vi "Autonomous Independent.vi"() -> ()   [LabVIEW 2016]
doc: "This VI is called when autonomous begins, and will automatically be terminated when autonomous ends. You can carry out timed or sensor driven robot movement independently without needing to return to the caller."
uses:
  <vilib>/Rock Robotics/WPI/ThirdParty/Sensors/Pigeon IMU/CTRE_PigeonIMU_TareType.ctl
  <vilib>/Rock Robotics/WPI/ThirdParty/CanMotor/TalonSRX/WPI_CANTalonSRX_BrakeOverride.ctl
  <vilib>/Rock Robotics/WPI/ThirdParty/CanMotor/TalonSRX/WPI_CANTalonSRX_APIControlMode.ctl
  Robot Global Data.vi
  <vilib>/Rock Robotics/Network Tables/NT Read Numeric Array.vi
  <vilib>/Rock Robotics/Network Tables/NT Write Number.vi
  <vilib>/Rock Robotics/Network Tables/NT Read String.vi
panel:
  in  "Disable Drive":bool
  in  "Norm":bool
  in  "Ms to top throttle":dbl=750.0 format="%#_13g"
  in  "Custom Sequence 2":cluster{"Values":dbl[], "Operation":u16[]}={"Values"=[0.0], "Operation"=[1000]} {"Operation" items=["Start"=0, "Drive Distance"=1, "Spin"=2, "Eject"=3, "Drive Time"=4, "Shoot Time"=5, "End"=1000, "Hold Position for ever"=1001]}
  in  "Custom Sequence 1":cluster{"Values":dbl[], "Operation":u16[]}={"Values"=[0.0], "Operation"=[1000]} {"Operation" items=["Start"=0, "Drive Distance"=1, "Spin"=2, "Eject"=3, "Drive Time"=4, "Shoot Time"=5, "End"=1000, "Hold Position for ever"=1001]}
  in  "Use Front Pannel":bool=TRUE
  in  "IZone":dbl=100.0
  in  "I":dbl=0.0125
  in  "Value to pass":dbl
  in  "Operation":i32
  in  "Start":bool
  in  "Go":bool
  in  "Case":i32
  in  "String":string="Nothing"
  in  "Rotate max throttle":dbl=0.666
  in  "Accept Error":dbl=1.0
  in  "F":dbl=0.11
  in  "P":dbl=0.0085
  in  "Acceptable Closed Loop error":dbl=0.01
  in  "Wheel Diameter":dbl=4.125
  in  "P":dbl=1.7
  in  "I":dbl
  in  "D":dbl=100.0
  in  "F":dbl=0.195
  in  "I Zone":dbl
  in  "Ramp Rate":dbl
  in  "P 2":dbl=1.7
  in  "I 2":dbl
  in  "D 2":dbl=100.0
  in  "F 2":dbl=0.195
  in  "I Zone 2":dbl
  in  "Ramp Rate 2":dbl
  # "Custom operation"
  # "Flow   Control"
  # "miscellaneous"
  # "Right"
  # "Left"
  # "Rotate"
  # "Drive Distance"
  # "Drive for time"
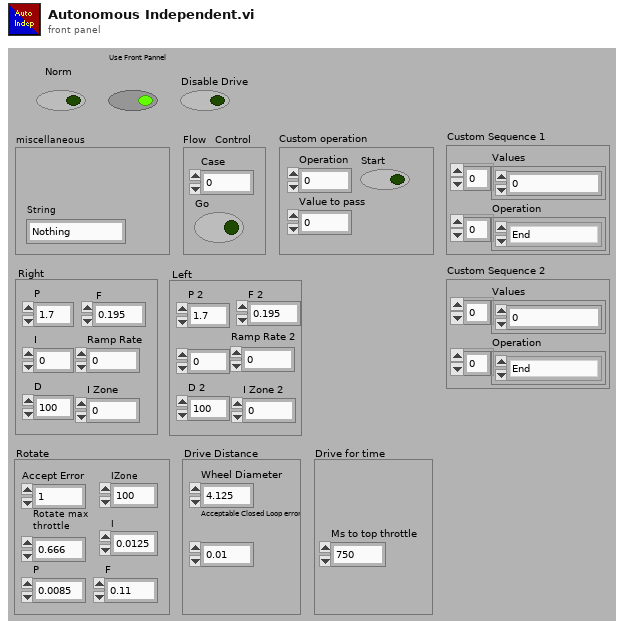
[diagram p1: front panel]
types:
  T1 = typedef "WPI_CANTalonSRX_BrakeOverride.ctl" = enum8{"No Override", "Override to Coast", "Override to Brake"}
  T2 = typedef "CTRE_PigeonIMU_TareType.ctl" = u8
  T3 = cluster{"P":dbl, "I":dbl, "D":dbl, "F":dbl, "IZone":dbl, "RampRate":dbl}
  T4 = enum16{"SOLID", "FLASH 500ms", "FLASH 1000ms", "OFF"}
  T5 = enum16{"OFF", "RED", "GREEN", "BLUE", "PURPLE", "YELLOW", "TEAL", "WHITE", "RAINBOW"}
  T6 = typedef "CTRE_PigeonIMU_DeviceRef.ctl" = cluster{"DeviceStatus":errorcluster, "Device Number":u8, "Type":T7, "Device ID":u32}
  T7 = typedef "CTRE_PigeonIMU_ConnectionType.ctl" = u32
  T8 = typedef "CTRE_PigeonIMU_GlobalStatus.ctl" = cluster{"PigeonState":T9, "FusedHeading":cluster{"Heading":dbl, "Valid?":bool, "Fusing?":bool}, "YPR":cluster{"Yaw":dbl, "Pitch":dbl, "Roll":dbl}, "Compass":cluster{"Heading":dbl, "Magnitude":dbl, "Absolute Heading":dbl}, "Accelerometer":cluster{"Biased":cluster{"X":i16, "Y":i16, "Z":i16, "Norm":i16}, "Angles":cluster{"XZ Tilt":dbl, "YZ Tilt":dbl, "XY Tilt":dbl}}, "Magnetometer":cluster{"Raw":cluster{"X":i16, "Y":i16, "Z":i16}, "Biased":cluster{"X":i16, "Y":i16, "Z":i16}}, "Gyro":cluster{"X":dbl, "Y":dbl, "Z":dbl, "Norm":dbl}, "6D Quaternian":cluster{"W":dbl, "X":dbl, "Y":dbl, "Z":dbl}, "Temp. (C)":dbl, "UpTime":u32, "StartupStatus":cluster{"ResetCount":i32, "ResetFlags":i32, "FirmwareVersion":i32, "HasReset?":bool}, "Calibration":cluster{"CurrentMode":T10, "LastCalError":i32, "CalBooting?":bool}, "CAN Error":errorcluster, "AccumGyro":cluster{"X":dbl, "Y":dbl, "Z":dbl}, "Usage Frame":u32}
  T9 = typedef "CTRE_PigeonIMU_PigeonState.ctl" = enum16{"NoComm", "Initializing", "Ready", "UserCalibration"}
  T10 = typedef "CTRE_PigeonIMU_CalibrationMode.ctl" = u16
  T11 = typedef "WPI_MotorControlDeviceRef.ctl" = cluster{"DeviceStatus":errorcluster, "Type":T12, "PWM":cluster{"PWM Channel":T13, "DeadBand":T14}, "CAN":cluster{"Device Number":u8, "SetOutput VI Ref":variant, "GetOutput VI Ref":variant, "Enable VI Ref":variant, "Disable VI Ref":variant, "Data":variant}, "Invert":bool}
  T12 = typedef "WPI_MotorControlType.ctl" = enum16{"PWM", "CAN"}
  T13 = typedef "FPGA_DIOPWMChannel.ctl" = enum8{"PWM 0", "PWM 1", "PWM 2", "PWM 3", "PWM 4", "PWM 5", "PWM 6", "PWM 7", "PWM 8", "PWM 9", "PWM MXP 0", "PWM MXP 1", "PWM MXP 2", "PWM MXP 3", "PWM MXP 4", "PWM MXP 5", "PWM MXP 6", "PWM MXP 7", "PWM MXP 8", "PWM MXP 9", "Invalid"}
  T14 = typedef "WPI_PWMDeadband.ctl" = cluster{"Name":string, "maxPositivePwm":i32, "minPositivePwm":i32, "centerPwm":i32, "maxNegativePwm":i32, "minNegativePwm":i32, "angularRange":u16}
  T15 = typedef "WPI_ServoDeviceRef.ctl" = cluster{"DeviceStatus":errorcluster, "PWM Channel":T13, "DeadBand":T14}
  T16 = typedef "WPI_CANTalonSRX_GlobalStatus.ctl" = cluster{"Applied Throttle":dbl, "Module Enabled":bool, "CAN Error":errorcluster, "Closed Loop Error":dbl, "Forward Limit Switch Closed":bool, "Reverse Limit Switch Closed":bool, "Sensor Position":dbl, "Sensor Velocity":dbl, "Current":dbl, "Sticky Fault - Over Temp":bool, "Sticky Fault - Under Voltage":bool, "Sticky Fault - Forward Limit":bool, "Sticky Fault - Reverse Limit":bool, "Sticky Fault - Forward Soft Limit":bool, "Sticky Fault - Reverse Soft Limit":bool, "Brake is Enabled":bool, "Encoder Position":dbl, "Encoder Velocity":dbl, "Encoder Index Count":dbl, "Encoder A Pin State":bool, "Encoder B Pin State":bool, "Encoder Index Pin State":bool, "Analog In":dbl, "Analog In Velocity":dbl, "Temperature (C)":dbl, "Battery Voltage":dbl, "Control 5 Is Supported":bool, "Current Profile Slot Select":dbl, "Pos Div 8":bool, "Vel Div 4":bool, "Pulse Width Position":i32, "Pulse Width Velocity":i32, "Pulse Width Rise To Rise (us)":i32, "Pulse Width Rise To Fall (us)":i32, "Mot Prof Active Is Under Run":bool, "Mot Prof Active Has Under Run":bool, "Mot Prof Active Is Last":bool, "Mot Prof Active Velocity Only":bool, "Mot Prof Active Is Valid":bool, "Mot Prof Buffer Is Full":bool, "Mot Prof Active Profile Slot Select":i32, "Mot Prof NextID":i32, "Mot Prof Count":i32, "Mot Prof Active Velocity":dbl, "Mot Prof Active Position":dbl, "Mot Prof Output Enable":i32, "UsageFrame":u32, "Motion Magic Active Trajectory":cluster{"Velocity":dbl, "Position":dbl}}
  T17 = typedef "WPI_CANTalonSRX_APIControlMode.ctl" = enum8{"Percent VBus", "Speed", "Position", "Slave", "Unchanged / Invalid", "Voltage Compensation", "Current", "Motion Profile", "Motion Magic"}
  T18 = typedef "NetComm_AllianceStation.ctl" = enum16{"Red 1", "Red 2", "Red 3", "Blue 1", "Blue 2", "Blue 3"}
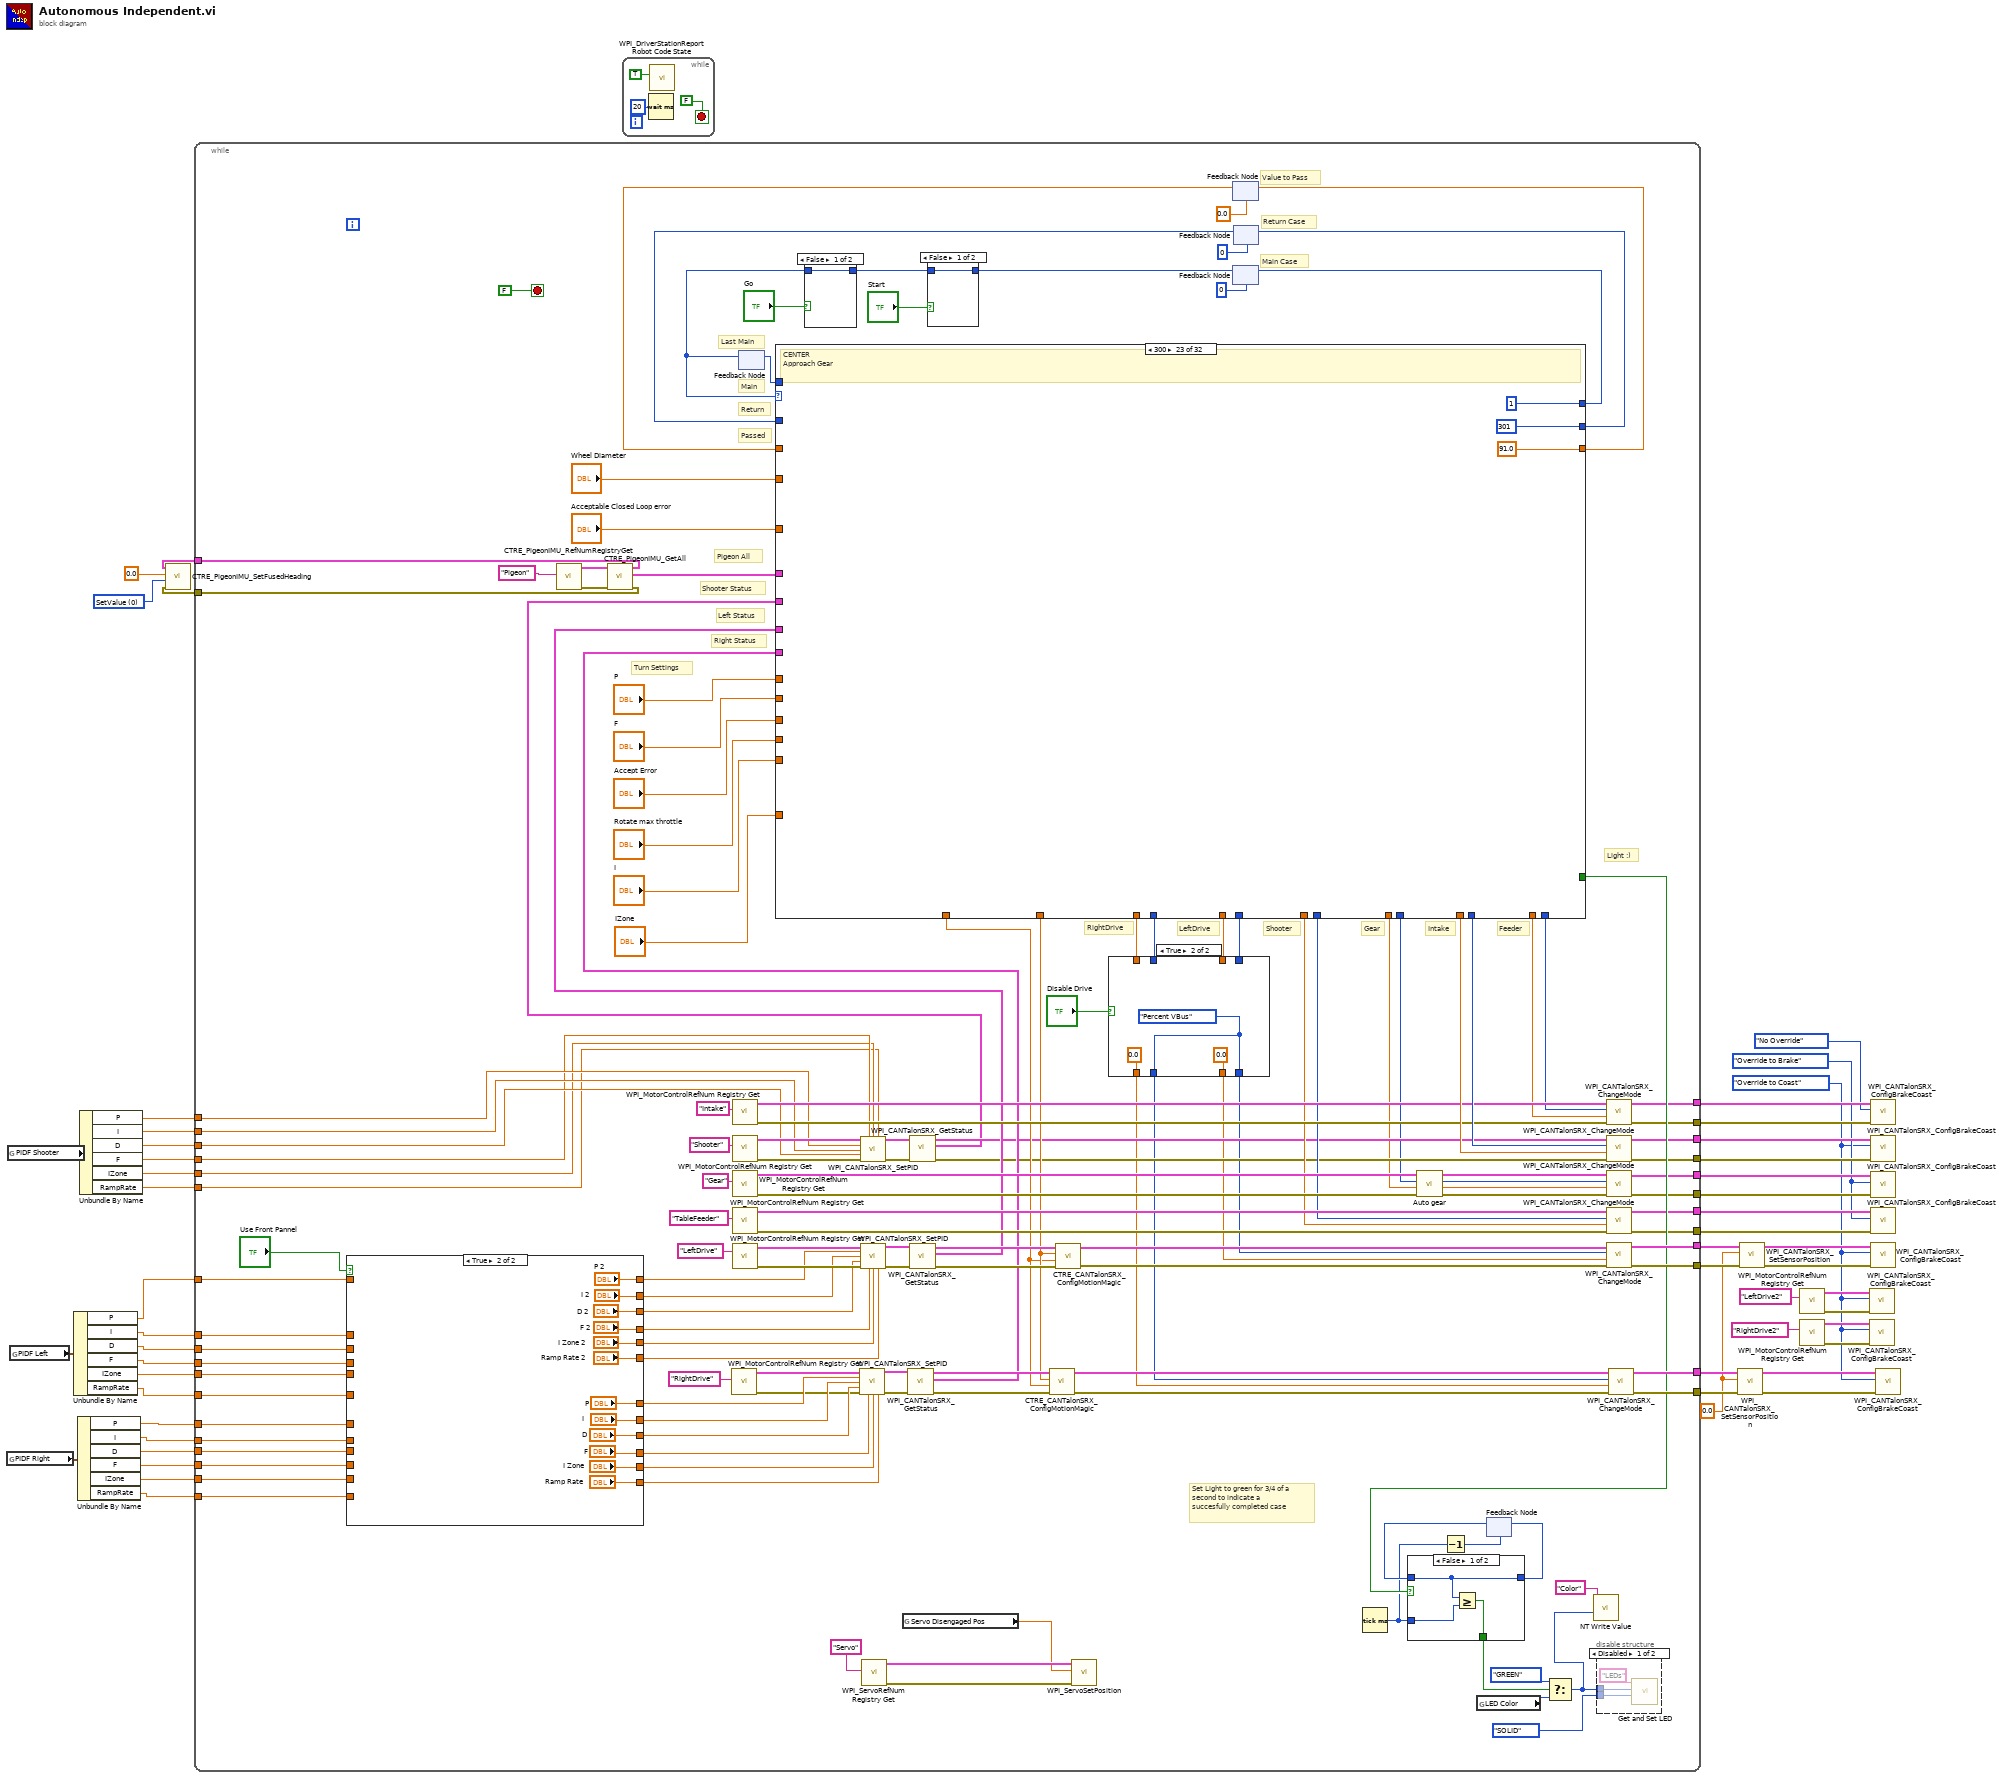
[diagram p0: block diagram]
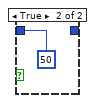
[diagram p5: hidden frame]
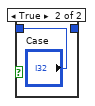
[diagram p6: hidden frame]
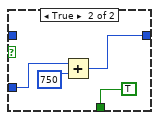
[diagram p7: hidden frame]
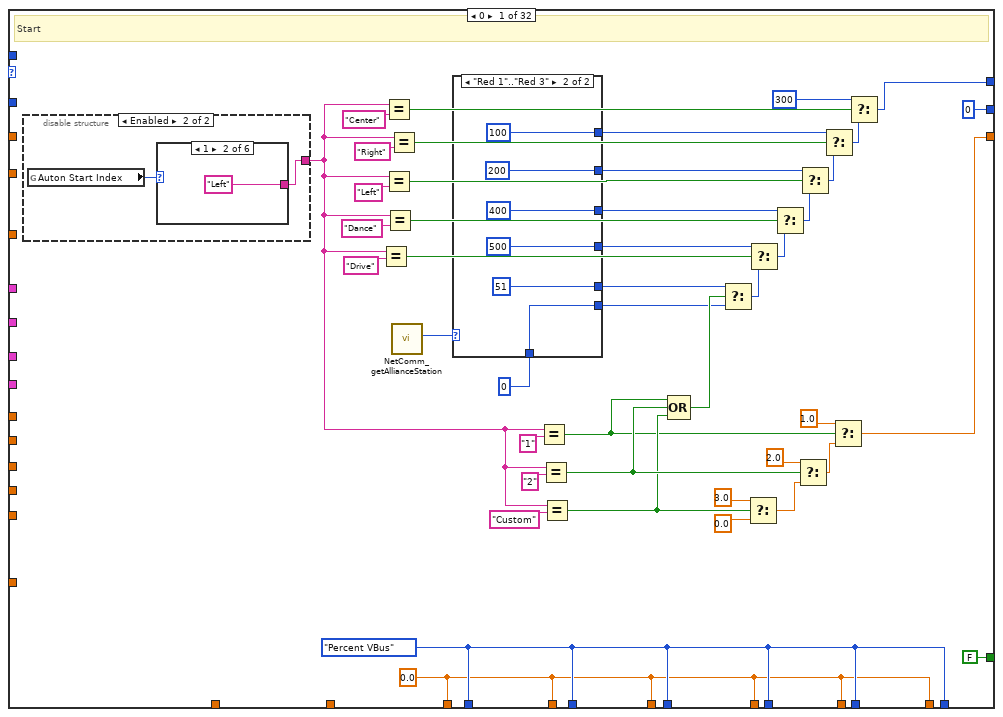
[diagram p8: hidden frame]
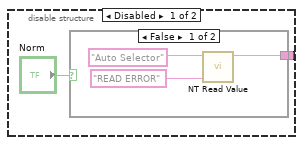
[diagram p9: hidden frame]
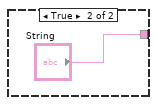
[diagram p10: hidden frame]
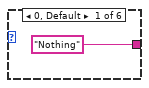
[diagram p11: hidden frame]
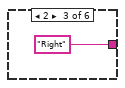
[diagram p12: hidden frame]
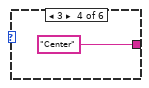
[diagram p13: hidden frame]
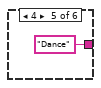
[diagram p14: hidden frame]
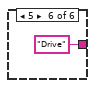
[diagram p15: hidden frame]
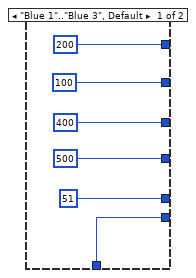
[diagram p16: hidden frame]
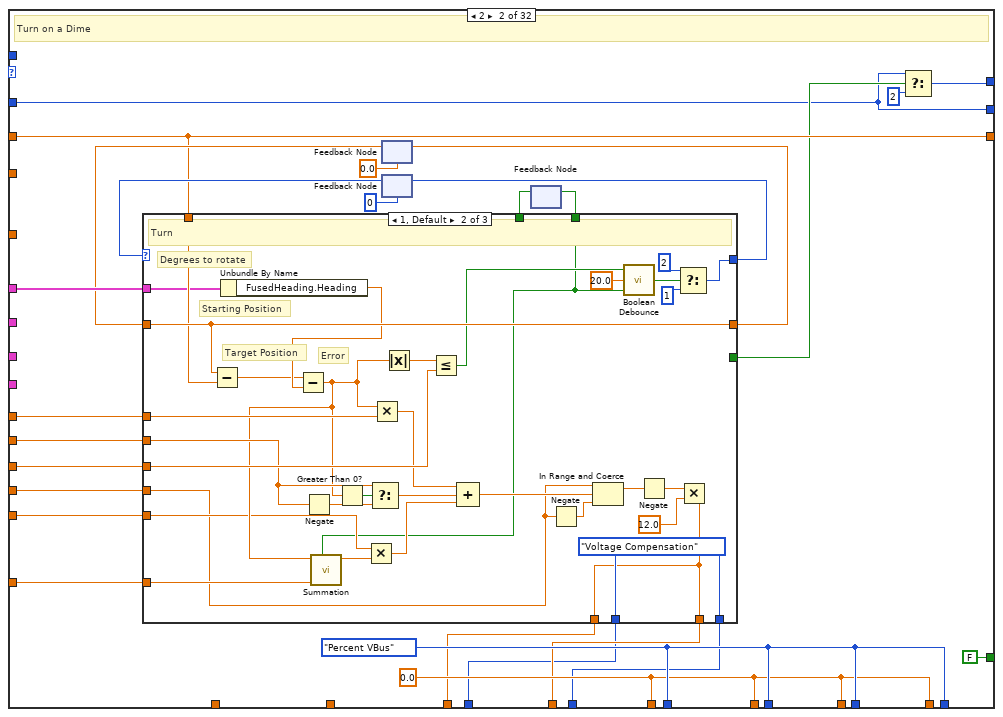
[diagram p17: hidden frame]
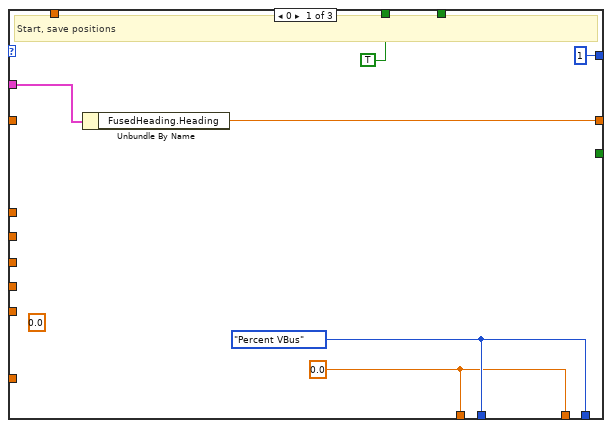
[diagram p18: hidden frame]
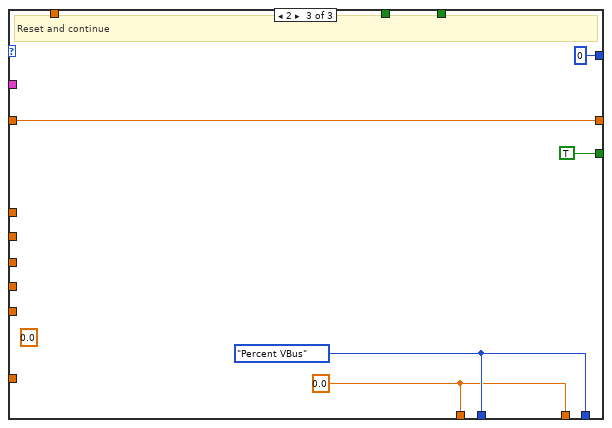
[diagram p19: hidden frame]
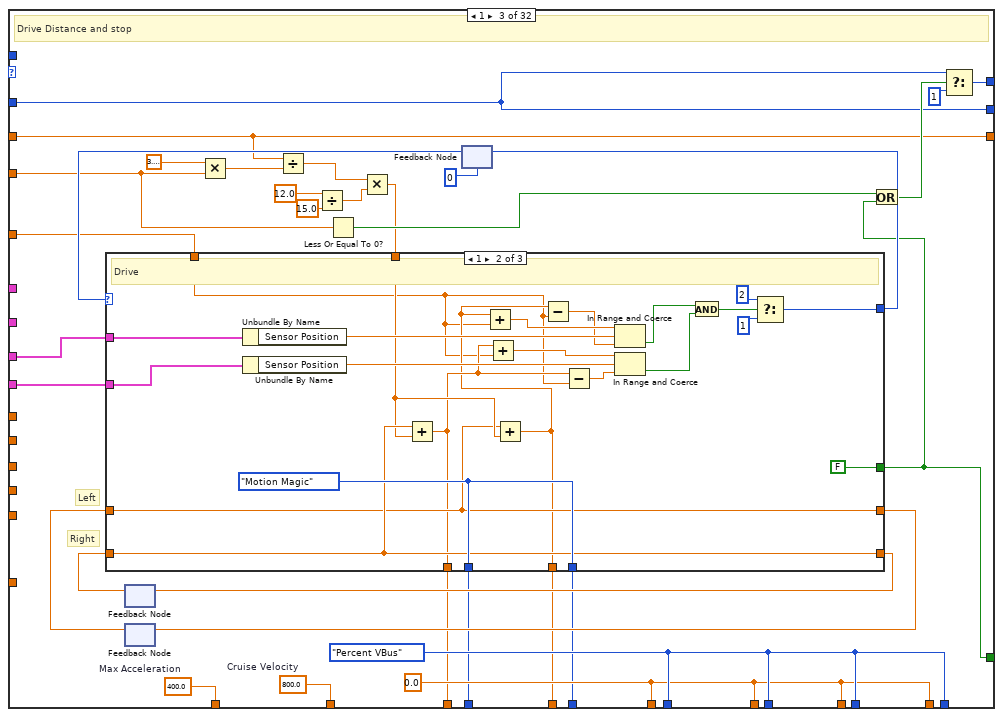
[diagram p20: hidden frame]
diagram:
  w8 = WPI_CANTalonSRX_BrakeOverride."Override to Brake" ("Brake / Coast Mode")
  w1 = WPI_CANTalonSRX_BrakeOverride."Override to Coast" ("Brake / Coast Mode")
  w46 = T2 0 items=["SetValue"=0, "AddOffset"=1, "MatchCompass"=2, "SetOffset"=255] ("TareType (SetValue)")
  w47 = 0.0 ("New Sensor Position")
  n1 = global read "Robot Global Data.vi" "PIDF Right"() -> (w42:T3)
  n2 = global read "Robot Global Data.vi" "PIDF Shooter"() -> (w22:T3)
  n3 = global read "Robot Global Data.vi" "PIDF Left"() -> (w41:T3)
  n4 = Unbundle By Name(w41) -> ("P"=w40:dbl, "I"=w39:dbl, "D"=w38:dbl, "F"=w37:dbl, "IZone"=w36:dbl, "RampRate"=w35:dbl)
  n5 = Unbundle By Name(w42) -> ("P"=w34:dbl, "I"=w33:dbl, "D"=w32:dbl, "F"=w31:dbl, "IZone"=w30:dbl, "RampRate"=w29:dbl)
  n6 = Unbundle By Name(w22) -> ("P"=w21:dbl, "I"=w20:dbl, "D"=w19:dbl, "F"=w18:dbl, "IZone"=w17:dbl, "RampRate"=w16:dbl)
  n7 = while {
    tunnel: [w153] -> w51
    tunnel: [w152] -> w50
    tunnel: [w151] -> w49
    tunnel: [w150] -> w48
    tunnel: [w119] -> w45
    tunnel: [w118] -> w44
    tunnel: w40 -> [w112]
    tunnel: w39 -> [w111]
    tunnel: w38 -> [w110]
    tunnel: w37 -> [w109]
    tunnel: w36 -> [w108]
    tunnel: w35 -> [w107]
    tunnel: w34 -> [w106]
    tunnel: w33 -> [w105]
    tunnel: w32 -> [w104]
    tunnel: w31 -> [w103]
    tunnel: w30 -> [w102]
    tunnel: w29 -> [w101]
    tunnel: [w97] -> w24
    tunnel: [w96] -> w23
    tunnel: w21 -> [w94]
    tunnel: w20 -> [w93]
    tunnel: w19 -> [w92]
    tunnel: w18 -> [w91]
    tunnel: w17 -> [w90]
    tunnel: w16 -> [w89]
    tunnel: [w86] -> w15
    tunnel: [w85] -> w14
    tunnel: [w84] -> w13
    tunnel: [w83] -> w12
    tunnel: [w82] -> w11
    tunnel: [w81] -> w10
    stop <- FALSE stop-if-true
    # "Last Main"
    # "Shooter Status"
    # "Main"
    # "Turn Settings"
    # "Return"
    # "Passed"
    # "Set Light to green for 3/4 of a second to indicate a succesfully completed case"
    # "Value to Pass"
    # "Main Case"
    # "Return Case"
    # "Feeder"
    # "Light :)"
    # "Intake"
    # "Gear"
    # "Shooter"
    # "LeftDrive"
    # "RightDrive"
    # "Pigeon All"
    # "Left Status"
    # "Right Status"
    n8 = case shown="True" "Use Front Pannel" {
      tunnel: [w213 "Ramp Rate 2"] -> w193
      tunnel: [w214 "I Zone 2"] -> w189
      tunnel: [w215 "F 2"] -> w188
      tunnel: [w216 "D 2"] -> w187
      tunnel: [w217 "I 2"] -> w186
      tunnel: [w218 "P 2"] -> w185
      tunnel: [w212 "P"] -> w180
      tunnel: [w211 "I"] -> w179
      tunnel: [w210 "D"] -> w178
      tunnel: [w209 "F"] -> w177
      tunnel: [w208 "I Zone"] -> w176
      tunnel: [w207 "Ramp Rate"] -> w175
      tunnel: w112 -> [w218 _]
      tunnel: w111 -> [w217 _]
      tunnel: w110 -> [w216 _]
      tunnel: w109 -> [w215 _]
      tunnel: w108 -> [w214 _]
      tunnel: w107 -> [w213 _]
      tunnel: w106 -> [w212 _]
      tunnel: w105 -> [w211 _]
      tunnel: w104 -> [w210 _]
      tunnel: w103 -> [w209 _]
      tunnel: w102 -> [w208 _]
      tunnel: w101 -> [w207 _]
      frame False {
      }
      frame True {
      }
    }
    n9 = call <vilib>:"CTRE_PigeonIMU_RefNumRegistryGet.vi"("refnum name"="Pigeon") -> ("error out"=w161:errorcluster, "PigeonIMUDevRef"=w162:T6)  [unwired: 9 in]
    n10 = call <vilib>:"CTRE_PigeonIMU_GetAll.vi"("error in (no error)"=w161, "PigeonIMUDevRef"=w162) -> ("error out"=w118:errorcluster, "Get All"=w196:T8, "PigeonIMUDevRef"=w119:T6)  [unwired: 7 in]
    n11 = call <vilib>:"WPI_MotorControlRefNum Registry Get.vi"("refnum name"="RightDrive") -> ("error out"=w173:errorcluster, "MotorControlDevRef"=w174:T11)  [unwired: 9 in]
    n12 = call <vilib>:"WPI_MotorControlRefNum Registry Get.vi"("refnum name"="Intake") -> ("error out"=w147:errorcluster, "MotorControlDevRef"=w148:T11)  [unwired: 9 in]
    n13 = call <vilib>:"WPI_MotorControlRefNum Registry Get.vi"("refnum name"="Shooter") -> ("error out"=w73:errorcluster, "MotorControlDevRef"=w167:T11)  [unwired: 9 in]
    n14 = call <vilib>:"WPI_MotorControlRefNum Registry Get.vi"("refnum name"="Gear") -> ("error out"=w169:errorcluster, "MotorControlDevRef"=w168:T11)  [unwired: 9 in]
    n15 = call <vilib>:"WPI_MotorControlRefNum Registry Get.vi"("refnum name"="TableFeeder") -> ("error out"=w171:errorcluster, "MotorControlDevRef"=w170:T11)  [unwired: 9 in]
    n16 = call <vilib>:"WPI_MotorControlRefNum Registry Get.vi"("refnum name"="LeftDrive") -> ("error out"=w190:errorcluster, "MotorControlDevRef"=w191:T11)  [unwired: 9 in]
    n17 = feedback #1() -> (w87:i32)  [unwired: 1 in]
    n18 = call <vilib>:"WPI_CANTalonSRX_SetPID.vi"("CAN Talon SRX Ref"=w174, "P"=w180, "I"=w179, "D"=w178, "error in (no error)"=w173, "F"=w177, "I Zone"=w176, "Ramp Rate"=w175) -> ("CAN Talon SRX Ref"=w181:T11, "error out"=w182:errorcluster)  [unwired: 6 in]
    n19 = call <vilib>:"WPI_CANTalonSRX_SetPID.vi"("CAN Talon SRX Ref"=w167, "P"=w94, "I"=w93, "D"=w92, "error in (no error)"=w73, "F"=w91, "I Zone"=w90, "Ramp Rate"=w89) -> ("CAN Talon SRX Ref"=w95:T11, "error out"=w74:errorcluster)  [unwired: 6 in]
    n20 = call <vilib>:"WPI_CANTalonSRX_SetPID.vi"("CAN Talon SRX Ref"=w191, "P"=w185, "I"=w186, "D"=w187, "error in (no error)"=w190, "F"=w188, "I Zone"=w189, "Ramp Rate"=w193) -> ("CAN Talon SRX Ref"=w192:T11, "error out"=w184:errorcluster)  [unwired: 6 in]
    n21 = call <vilib>:"WPI_ServoRefNum Registry Get.vi"("refnum name"="Servo") -> ("error out"=w62:errorcluster, "ServoDeviceRef"=w63:T15)  [unwired: 9 in]
    n22 = global read "Robot Global Data.vi" "Servo Disengaged Pos"() -> (w52:dbl)
    n23 = call <vilib>:"WPI_CANTalonSRX_GetStatus.vi"("error in (no error)"=w182, "CAN Talon SRX Ref"=w181) -> ("error out"=w137:errorcluster, "Talon SRX Status"=w120:T16, "CAN Talon SRX Ref"=w138:T11)  [unwired: 7 in]
    n24 = call <vilib>:"WPI_CANTalonSRX_GetStatus.vi"("error in (no error)"=w74, "CAN Talon SRX Ref"=w95) -> ("error out"=w99:errorcluster, "Talon SRX Status"=w98:T16, "CAN Talon SRX Ref"=w100:T11)  [unwired: 7 in]
    n25 = call <vilib>:"WPI_CANTalonSRX_GetStatus.vi"("error in (no error)"=w184, "CAN Talon SRX Ref"=w192) -> ("error out"=w139:errorcluster, "Talon SRX Status"=w121:T16, "CAN Talon SRX Ref"=w140:T11)  [unwired: 7 in]
    n26 = call <vilib>:"WPI_ServoSetPosition.vi"("error in (no error)"=w62, "Position"=w52, "ServoDeviceRef"=w63) -> ()  [unwired: 7 in, 2 out]
    n27 = feedback #2(0.0) -> (w155:dbl)
    n28 = feedback #3(0) -> (w80:i32)
    n29 = case shown="False" "Start" {
      tunnel: w80 -> [w231 _]
      tunnel: [w231 50] -> w125
      frame False {
      }
      frame True {
      }
    }
    n30 = case shown="False" "Go" {
      tunnel: [w233 "Case"] -> w88
      tunnel: w125 -> [w233 _]
      frame False {
      }
      frame True {
      }
    }
    n31 = feedback-in #1(w88) -> ()
    n32 = feedback #4(0) -> (w160:i32)
    n33 = case shown="300" w88 {
      tunnel: [w284 w337 w412 w462 _ w617 _ _ _ _ _ _ _ _ _ _ _ _ _ _ _ _ _ _ _ _ _ _ _ _ _ w789] -> w194
      tunnel: [w283 w336 w411 w469 _ w607 _ _ _ _ _ _ _ _ _ _ _ _ _ _ _ _ _ _ _ _ _ _ _ _ _ w790] -> w195
      tunnel: [w284 w337 w412 w462 _ w617 _ _ _ _ _ _ _ _ _ _ _ _ _ _ _ _ _ _ _ _ _ _ _ _ _ w789] -> w77
      tunnel: [w283 w336 w411 -0.99 _ _ _ _ _ _ _ _ _ _ _ _ _ _ _ _ _ _ _ _ _ _ _ _ _ _ _ w790] -> w78
      tunnel: [w284 w337 w412 w462 _ w611 _ _ _ _ _ _ _ _ _ _ _ _ _ _ _ _ _ _ _ _ _ _ _ _ _ w789] -> w117
      tunnel: [w283 w336 w411 w469 _ w610 _ _ _ _ _ _ _ _ _ _ _ _ _ _ _ _ _ _ _ _ _ _ _ _ _ w790] -> w116
      tunnel: [w284 w335 w401 w463 w557 w617 _ _ _ _ _ _ _ _ _ _ _ _ _ _ _ _ _ _ _ _ _ _ _ _ _ w789] -> w70
      tunnel: [w283 w334 w400 w458 w548 _ _ _ _ _ _ _ _ _ _ _ _ _ _ _ _ _ _ _ _ _ _ _ _ _ _ w797] -> w72
      tunnel: [w284 w333 w402 w466 w557 w617 _ _ _ _ _ _ _ _ _ _ _ _ _ _ _ _ _ _ _ _ _ _ _ _ _ w789] -> w66
      tunnel: [w283 w332 w403 w460 w549 _ _ _ _ _ _ _ _ _ _ _ _ _ _ _ _ _ _ _ _ _ _ _ _ _ _ w796] -> w68
      tunnel: w196 -> [_ w327 _ _ w538 _ _ _ _ w695 _ _ _ w711 _ _ w724 _ _ _ w744 _ _ _ _ _ _ w770 w777 _ _ _]
      tunnel: w160 -> [_ w314 w393 w453 w564 w629 _ _ _ _ _ _ _ _ _ _ _ _ _ _ _ _ _ _ _ _ _ _ _ _ _ _]
      tunnel: [0 w314 w393 w453 w564 w629 1000 w657 101 103 103 104 105 106 1001 201 203 203 204 205 206 1001 301 1001 1001 401 403 403 402 1001 1000 1000] -> w159
      tunnel: [w242 w328 w415 w489 w565 w630 "Operation" w665 1 ("t") 2 ("t") 103 ("t") 1 ("t") 3 ("t") 2 ("t") 1 ("t") 1 ("t") 2 ("t") 203 ("t") 1 ("t") 3 ("t") 2 ("t") 1 ("t") 1 ("t") 3 ("t") 2 ("t") 1 ("t") 2 ("t") 2 ("t") 2 ("t") 1 ("t") 1000 ("t") 1001 ("t")] -> w79
      tunnel: [FALSE FALSE w399 w476 _ _ _ _ _ _ _ _ _ _ _ _ _ _ _ _ _ _ _ _ _ _ _ _ _ _ FALSE TRUE] -> w132
      tunnel: w155 -> [_ w323 w384 w477 w545 w619 _ w663 _ _ _ _ _ _ _ _ _ _ _ _ _ _ _ _ _ _ _ _ _ _ _ _]
      tunnel: [w248 w323 w384 w477 w545 w619 "Value to pass" w671 88.5 w692 0.0 27.5 -25.0 w710 144.0 ("Value to pass") 79.5 w726 0.0 ("Value to pass") 50.5 ("Value to pass") -25.0 w741 144.0 ("Value to pass") 91.0 ("Value to pass") -25.0 ("Value to pass") w756 20.0 ("Value to pass") 45.0 ("Value to pass") w771 w778 72.0 ("Value to pass") 0.0 0.0] -> w154
      tunnel: w121 -> [_ _ w414 w488 _ _ _ _ _ _ _ _ _ _ _ _ _ _ _ _ _ _ _ _ _ _ _ _ _ _ _ w801]
      tunnel: w120 -> [_ _ w413 w487 _ _ _ _ _ _ _ _ _ _ _ _ _ _ _ _ _ _ _ _ _ _ _ _ _ _ _ w800]
      tunnel: [w284 w337 w412 w462 _ w615 _ _ _ _ _ _ _ _ _ _ _ _ _ _ _ _ _ _ _ _ _ _ _ _ _ w789] -> w146
      tunnel: [w283 w336 w411 w469 _ w614 _ _ _ _ _ _ _ _ _ _ _ _ _ _ _ _ _ _ _ _ _ _ _ _ _ w790] -> w145
      tunnel: "Wheel Diameter" -> [_ _ w389 w478 _ _ _ _ _ _ _ _ _ _ _ _ _ _ _ _ _ _ _ _ _ _ _ _ _ _ _ _]
      tunnel: "Acceptable Closed Loop error" -> [_ _ w397 w472 _ _ _ _ _ _ _ _ _ _ _ _ _ _ _ _ _ _ _ _ _ _ _ _ _ _ _ _]
      tunnel: "P" -> [_ w322 _ _ _ _ _ _ _ _ _ _ _ _ _ _ _ _ _ _ _ _ _ _ _ _ _ _ _ _ _ _]
      tunnel: "F" -> [_ w321 _ _ _ _ _ _ _ _ _ _ _ _ _ _ _ _ _ _ _ _ _ _ _ _ _ _ _ _ _ _]
      tunnel: "Accept Error" -> [_ w320 _ _ _ _ _ _ _ _ _ _ _ _ _ _ _ _ _ _ _ _ _ _ _ _ _ _ _ _ _ _]
      tunnel: "Rotate max throttle" -> [_ w319 _ _ _ _ _ _ _ _ _ _ _ _ _ _ _ _ _ _ _ _ _ _ _ _ _ _ _ _ _ _]
      tunnel: [_ _ w394 w470 _ _ _ _ _ _ _ _ _ _ _ _ _ _ _ _ _ _ _ _ _ _ _ _ _ _ _ 850.0] -> w123
      tunnel: [_ _ w392 w467 _ _ _ _ _ _ _ _ _ _ _ _ _ _ _ _ _ _ _ _ _ _ _ _ _ _ _ 600.0] -> w122
      tunnel: "I" -> [_ w313 _ _ _ _ _ _ _ _ _ _ _ _ _ _ _ _ _ _ _ _ _ _ _ _ _ _ _ _ _ _]
      tunnel: "IZone" -> [_ w312 _ _ _ _ _ _ _ _ _ _ _ _ _ _ _ _ _ _ _ _ _ _ _ _ _ _ _ _ _ _]
      tunnel: w98 -> [_ _ _ _ _ w609 _ _ _ _ _ _ _ _ _ _ _ _ _ _ _ _ _ _ _ _ _ _ _ _ _ _]
      tunnel: w87 -> [_ _ _ _ _ _ _ w666 _ _ _ _ _ _ _ _ _ _ _ _ _ _ _ _ _ _ _ _ _ _ _ w803]
      frame 0 {
        w283 = 0.0
        w284 = WPI_CANTalonSRX_APIControlMode."Percent VBus" ("Control Mode")
        # "Start"
        n34 = disable-structure shown="Enabled" {
          disable-tunnel: [w287 w292] -> w243
          frame Disabled {
            n35 = case shown="False" "Norm" {
              tunnel: [w289 "String"] -> w287
              frame False {
                n36 = call-poly <vilib>:"NT Read Value.vi"("Default Value"="READ ERROR", "Name"="Auto Selector") -> ("String"=w289:string)  [unwired: 8 in, 1 out]
              }
              frame True {
              }
            }
          }
          frame Enabled {
            n37 = global read "Robot Global Data.vi" "Auton Start Index"() -> (w293:i32)
            n38 = case shown="1" w293 {
              tunnel: ["Nothing" ("y") "Left" ("y") "Right" ("y") "Center" ("y") "Dance" ("y") "Drive" ("y")] -> w292
              frame 0, Default {
              }
              frame 1 {
              }
              frame 2 {
              }
              frame 3 {
              }
              frame 4 {
              }
              frame 5 {
              }
            }
          }
        }
        n39 = Equal?(x=w243, y="Drive") -> (x = y?=w265:bool)
        n40 = Equal?(x=w243, y="Center") -> (x = y?=w276:bool)
        n41 = Equal?(x=w243, y="Left") -> (x = y?=w279:bool)
        n42 = Equal?(x=w243, y="Dance") -> (x = y?=w269:bool)
        n43 = Equal?(x=w243, y="Right") -> (x = y?=w275:bool)
        n44 = call <vilib>:"NetComm_getAllianceStation.vi"() -> ("Alliance Station"=w262:T18)  [unwired: 10 in, 1 out]
        n45 = case shown="\"Red 1\"..\"Red 3\"" w262 {
          tunnel: [200 100] -> w273
          tunnel: [100 200] -> w272
          tunnel: [400 ("t") 400 ("t")] -> w268
          tunnel: [500 ("t") 500 ("t")] -> w266
          tunnel: [51 ("t") 51 ("f")] -> w259
          tunnel: 0 ("f") -> [w300 w306]
          tunnel: [w300 w306] -> w244
          frame "Blue 1".."Blue 3", Default {
          }
          frame "Red 1".."Red 3" {
          }
        }
        n46 = Equal?(x=w243, y="1") -> (x = y?=w250:bool)
        n47 = Equal?(x=w243, y="2") -> (x = y?=w252:bool)
        n48 = Equal?(x=w243, y="Custom") -> (x = y?=w251:bool)
        n49 = Compound Arithmetic op=OR(w250, w252, w251) -> (w255:bool)
        n50 = Select(t=w259, s=w255, f=w244) -> (s? t:f=w260:i32)
        n51 = Select(t=3.0, s=w251, f=0.0) -> (s? t:f=w254:dbl)
        n52 = Select(t=w266, s=w265, f=w260) -> (s? t:f=w263:i32)
        n53 = Select(t=w268, s=w269, f=w263) -> (s? t:f=w270:i32)
        n54 = Select(t=2.0, s=w252, f=w254) -> (s? t:f=w253:dbl)
        n55 = Select(t=w272, s=w279, f=w270) -> (s? t:f=w278:i32)
        n56 = Select(t=w273, s=w275, f=w278) -> (s? t:f=w277:i32)
        n57 = Select(t=1.0, s=w250, f=w253) -> (s? t:f=w248:dbl)
        n58 = Select(t=300, s=w276, f=w277) -> (s? t:f=w242:i32)
      }
      frame 2 {
        w336 = 0.0
        w337 = WPI_CANTalonSRX_APIControlMode."Percent VBus" ("Control Mode")
        # "Turn on a Dime"
        n59 = feedback #5(0.0) -> (w324:dbl)
        n60 = feedback #6(0) -> (w331:i32)
        n61 = feedback #7() -> (w315:bool)  [unwired: 1 in]
        n62 = case shown="1, Default" w331 {
          tunnel: [w342 w377 w380] -> w335
          tunnel: [w341 w354 w379] -> w334
          tunnel: [w342 w377 w380] -> w333
          tunnel: [w341 w354 w379] -> w332
          tunnel: [1 w373 0] -> w329
          tunnel: w327 -> [w344 w372 _]
          tunnel: [w343 w376 w381] -> w325
          tunnel: w324 -> [_ w376 w381]
          tunnel: w323 -> [_ w375 _]
          tunnel: w322 -> [_ w374 _]
          tunnel: w321 -> [_ w364 _]
          tunnel: w320 -> [_ w367 _]
          tunnel: w319 -> [_ w351 _]
          tunnel: [_ _ TRUE] -> w317
          tunnel: [TRUE _ _] -> w316
          tunnel: w315 -> [_ w345 _]
          tunnel: w313 -> [_ w357 _]
          tunnel: w312 -> [_ w358 _]
          frame 0 {
            (unwired) 0.0
            w341 = 0.0
            w342 = WPI_CANTalonSRX_APIControlMode."Percent VBus" ("Control Mode")
            # "Start, save positions"
            n63 = Unbundle By Name(w344) -> ("FusedHeading.Heading"=w343:dbl)
          }
          frame 1, Default {
            w377 = WPI_CANTalonSRX_APIControlMode."Voltage Compensation" ("Control Mode")
            # "Error"
            # "Starting Position"
            # "Degrees to rotate"
            # "Target Position"
            # "Turn"
            n64 = Subtract(x=w376, y=w375) -> (x-y=w370:dbl)
            n65 = Unbundle By Name(w372) -> ("FusedHeading.Heading"=w371:dbl)
            n66 = Subtract(x=w370, y=w371) -> (x-y=w359:dbl)
            n67 = Negate(x=w364) -> (-x=w363:dbl)
            n68 = call "Summation.vi"("Reset"=w345, "Zone"=w358, "Number"=w359) -> ("sum"=w356:dbl)  [unwired: 8 in]
            n69 = Greater Than 0?(x=w359) -> (x > 0?=w365:bool)
            n70 = Multiply(x=w357, y=w356) -> (x*y=w355:dbl)
            n71 = Select(t=w364, s=w365, f=w363) -> (s? t:f=w360:dbl)
            n72 = Multiply(x=w359, y=w374) -> (x*y=w361:dbl)
            n73 = Absolute Value(x=w359) -> (abs(x)=w368:dbl)
            n74 = Less Or Equal?(x=w368, y=w367) -> (x <= y?=w347:bool)
            n75 = Compound Arithmetic op=ADD(w361, w360, w355) -> (w353:dbl)
            n76 = Negate(x=w351) -> (-x=w352:dbl)
            n77 = In Range and Coerce(upper limit=w351, x=w353, lower limit=w352) -> (coerced(x)=w350:dbl)  [unwired: 1 out]
            n78 = call "Boolean Debounce.vi"("Reset"=w345, "Miliseconds"=20.0 ("Cycles"), "In"=w347) -> ("Debounced"=w348:bool)
            n79 = Negate(x=w350) -> (-x=w349:dbl)
            n80 = Select(t=2, s=w348, f=1) -> (s? t:f=w373:i32)
            n81 = Multiply(x=w349, y=12.0) -> (x*y=w354:dbl)
          }
          frame 2 {
            (unwired) 0.0
            w379 = 0.0
            w380 = WPI_CANTalonSRX_APIControlMode."Percent VBus" ("Control Mode")
            # "Reset and continue"
          }
        }
        n82 = feedback-in #5(w325) -> ()
        n83 = feedback-in #6(w329) -> ()
        n84 = feedback-in #7(w316) -> ()
        n85 = Select(t=w314, s=w317, f=2) -> (s? t:f=w328:i32)
      }
      frame 1 {
        w392 = 400.0  # Max Acceleration
        w394 = 800.0  # Cruise Velocity
        w411 = 0.0
        w412 = WPI_CANTalonSRX_APIControlMode."Percent VBus" ("Control Mode")
        # "Right"
        # "Left"
        # "Drive Distance and stop"
        n86 = feedback #8() -> (w406:dbl)  [unwired: 1 in]
        n87 = feedback #9() -> (w404:dbl)  [unwired: 1 in]
        n88 = Multiply(x=3.141592653589793, y=w389) -> (x*y=w383:dbl)
        n89 = Divide(x=w384, y=w383) -> (x/y=w391:dbl)
        n90 = Divide(x=12.0, y=15.0) -> (x/y=w387:dbl)
        n91 = Less Or Equal To 0?(x=w389) -> (x <= 0?=w398:bool)
        n92 = Multiply(x=w391, y=w387) -> (x*y=w388:dbl)
        n93 = feedback #10(0) -> (w410:i32)
        n94 = case shown="1" w410 {
          tunnel: w414 -> [w423 w444 _]
          tunnel: w413 -> [w422 w443 _]
          tunnel: [1 w437 0] -> w408
          tunnel: [w420 w432 0.0 ("Sensor Position")] -> w405
          tunnel: [w419 w438 0.0 ("Sensor Position")] -> w407
          tunnel: w406 -> [_ w438 _]
          tunnel: w404 -> [_ w432 _]
          tunnel: [w417 w429 w448] -> w403
          tunnel: [w418 w445 w449] -> w402
          tunnel: [w418 w445 w449] -> w401
          tunnel: [w417 w427 w448] -> w400
          tunnel: [FALSE FALSE TRUE] -> w399
          tunnel: w388 -> [_ w433 _]
          tunnel: w397 -> [_ w426 _]
          frame 0, Default {
            w417 = 0.0
            w418 = WPI_CANTalonSRX_APIControlMode."Percent VBus" ("Control Mode")
            # "Record Sensor Position"
            n95 = Unbundle By Name(w423) -> ("Sensor Position"=w420:dbl)
            n96 = Unbundle By Name(w422) -> ("Sensor Position"=w419:dbl)
          }
          frame 1 {
            w445 = WPI_CANTalonSRX_APIControlMode."Motion Magic" ("Control Mode")
            # "Drive"
            n97 = Unbundle By Name(w444) -> ("Sensor Position"=w442:dbl)
            n98 = Unbundle By Name(w443) -> ("Sensor Position"=w434:dbl)
            n99 = Add(x=w438, y=w433) -> (x+y=w429:dbl)
            n100 = Add(x=w429, y=w426) -> (x+y=w430:dbl)
            n101 = Add(x=w432, y=w433) -> (x+y=w427:dbl)
            n102 = Add(x=w427, y=w426) -> (x+y=w431:dbl)
            n103 = Subtract(x=w427, y=w426) -> (x-y=w425:dbl)
            n104 = Subtract(x=w429, y=w426) -> (x-y=w428:dbl)
            n105 = In Range and Coerce(upper limit=w431, x=w442, lower limit=w425) -> (In Range?=w441:bool)  [unwired: 1 out]
            n106 = In Range and Coerce(upper limit=w430, x=w434, lower limit=w428) -> (In Range?=w440:bool)  [unwired: 1 out]
            n107 = And(x=w441, y=w440) -> (x .and. y?=w424:bool)
            n108 = Select(t=2, s=w424, f=1) -> (s? t:f=w437:i32)
          }
          frame 2 {
            w448 = 0.0
            w449 = WPI_CANTalonSRX_APIControlMode."Percent VBus" ("Control Mode")
            # "Finish and reset"
          }
        }
        n109 = feedback-in #8(w407) -> ()
        n110 = feedback-in #9(w405) -> ()
        n111 = feedback-in #10(w408) -> ()
        n112 = Or(x=w398, y=w399) -> (x .or. y?=w396:bool)
        n113 = Select(t=w393, s=w396, f=1) -> (s? t:f=w415:i32)
      }
      frame 3 {
        w467 = 80.0  # Max Acceleration
        w470 = 290.0  # Cruise Velocity
        w469 = 0.0
        w462 = WPI_CANTalonSRX_APIControlMode."Percent VBus" ("Control Mode")
        # "Right"
        # "Left"
        # "Drive Distance while ejecting gear then stop"
        n114 = feedback #11() -> (w482:dbl)  [unwired: 1 in]
        n115 = feedback #12() -> (w480:dbl)  [unwired: 1 in]
        n116 = Multiply(x=3.141592653589793, y=w478) -> (x*y=w473:dbl)
        n117 = Divide(x=w477, y=w473) -> (x/y=w475:dbl)
        n118 = Less Or Equal To 0?(x=w473) -> (x <= 0?=w474:bool)
        n119 = feedback #13(0) -> (w486:i32)
        n120 = case shown="2" w486 {
          tunnel: w488 -> [w505 w527 _]
          tunnel: w487 -> [w504 w526 _]
          tunnel: [1 w520 0] -> w484
          tunnel: [w502 w515 0.0 ("Sensor Position")] -> w481
          tunnel: [w501 w521 0.0 ("Sensor Position")] -> w483
          tunnel: w482 -> [_ w521 _]
          tunnel: w480 -> [_ w515 _]
          tunnel: [w499 w512 w532] -> w461
          tunnel: [w500 w528 w533] -> w465
          tunnel: [w500 w528 w533] -> w464
          tunnel: [w499 w510 w532] -> w459
          tunnel: [FALSE FALSE TRUE] -> w476
          tunnel: w475 -> [_ w516 _]
          tunnel: w472 -> [_ w509 _]
          tunnel: [TRUE ("Reset") FALSE ("Reset") TRUE ("Reset")] -> w457
          frame 0, Default {
            w499 = 0.0
            w500 = WPI_CANTalonSRX_APIControlMode."Percent VBus" ("Control Mode")
            # "Record Sensor Position"
            n121 = Unbundle By Name(w504) -> ("Sensor Position"=w501:dbl)
            n122 = Unbundle By Name(w505) -> ("Sensor Position"=w502:dbl)
          }
          frame 1 {
            w528 = WPI_CANTalonSRX_APIControlMode."Motion Magic" ("Control Mode")
            # "Drive"
            n123 = Unbundle By Name(w527) -> ("Sensor Position"=w525:dbl)
            n124 = Unbundle By Name(w526) -> ("Sensor Position"=w517:dbl)
            n125 = Add(x=w521, y=w516) -> (x+y=w512:dbl)
            n126 = Add(x=w512, y=w509) -> (x+y=w513:dbl)
            n127 = Add(x=w515, y=w516) -> (x+y=w510:dbl)
            n128 = Add(x=w510, y=w509) -> (x+y=w514:dbl)
            n129 = Subtract(x=w510, y=w509) -> (x-y=w508:dbl)
            n130 = Subtract(x=w512, y=w509) -> (x-y=w511:dbl)
            n131 = In Range and Coerce(upper limit=w514, x=w525, lower limit=w508) -> (In Range?=w524:bool)  [unwired: 1 out]
            n132 = In Range and Coerce(upper limit=w513, x=w517, lower limit=w511) -> (In Range?=w523:bool)  [unwired: 1 out]
            n133 = And(x=w524, y=w523) -> (x .and. y?=w507:bool)
            n134 = Select(t=2, s=w507, f=1) -> (s? t:f=w520:i32)
          }
          frame 2 {
            w532 = 0.0
            w533 = WPI_CANTalonSRX_APIControlMode."Percent VBus" ("Control Mode")
            # "Finish and reset"
          }
        }
        n135 = feedback-in #11(w483) -> ()
        n136 = feedback-in #12(w481) -> ()
        n137 = call "ms.vi"("Reset"=w457) -> ("millisecond"=w455:u32)
        n138 = Greater?(x=w455, y=u32 750) -> (0:w454:bool)
        n139 = case shown="False" w454 {
          tunnel: [w492 w496] -> w466
          tunnel: w465 -> [_ w496]
          tunnel: w464 -> [_ w495]
          tunnel: [w492 w495] -> w463
          tunnel: w462 -> [w492 _]
          tunnel: w461 -> [_ w493]
          tunnel: [0.0 w493] -> w460
          tunnel: w459 -> [_ w494]
          tunnel: [0.0 w494] -> w458
          frame False {
          }
          frame True {
          }
        }
        n140 = feedback-in #13(w484) -> ()
        n141 = Or(x=w474, y=w476) -> (x .or. y?=w452:bool)
        n142 = Select(t=w453, s=w452, f=3) -> (s? t:f=w489:i32)
      }
      frame 4 {
        w542 = 1.0  # Top Throttle
        w557 = WPI_CANTalonSRX_APIControlMode."Percent VBus" ("Control Mode")
        # "Drive for time with set acceleration acceleration/deceleration periond"
        n143 = Greater Than 0?(x=w545) -> (x > 0?=w546:bool)
        n144 = Negate(x=w542) -> (-x=w543:dbl)
        n145 = Select(t=w542, s=w546, f=w543) -> (s? t:f=w547:dbl)
        n146 = Absolute Value(x=w545) -> (abs(x)=w544:dbl)
        n147 = Multiply(x=w544, y=1000.0) -> (x*y=w556:dbl)
        n148 = feedback #14(TRUE) -> (w551:bool)
        n149 = feedback #15(0 ("f")) -> (w559:i32)
        n150 = feedback #16() -> (w536:dbl)  [unwired: 1 in]
        n151 = call "ms.vi"("Reset"=w551) -> ("millisecond"=w558:u32)
        n152 = case shown="1" w559 {
          tunnel: [FALSE FALSE TRUE] -> w562
          tunnel: [1 ("f") w588 0 ("f")] -> w561
          tunnel: w558 -> [_ w581 _]
          tunnel: [FALSE FALSE TRUE] -> w552
          tunnel: w556 -> [_ w583 _]
          tunnel: [0.0 w578 0.0] -> w553
          tunnel: w547 -> [_ w573 _]
          tunnel: w538 -> [w567 _ w602]
          tunnel: w536 -> [_ w572 _]
          tunnel: [w566 w572 w601] -> w537
          frame 0, Default {
            n153 = Unbundle By Name(w567) -> ("FusedHeading.Heading"=w566:dbl)
          }
          frame 1 {
            n154 = Divide(x=w583, y=2.0) -> (x/y=w575:dbl)
            n155 = Round To Nearest(number=w575) -> (nearest integer value=w576:dbl)
            n156 = Greater?(x=w581, y=w575) -> (0:w580:bool)
            n157 = case shown="True" w580 {
              tunnel: [w596 w597] -> w577
              tunnel: w581 -> [w596 w600]
              tunnel: w576 -> [_ w598]
              frame False {
              }
              frame True {
                n158 = Subtract(x=w600, y=w598) -> (x-y=w599:dbl)
                n159 = Subtract(x=w598, y=w599) -> (x-y=w597:dbl)
              }
            }
            n160 = Greater?(x=w577, y="Ms to top throttle") -> (0:w579:bool)
            n161 = case shown="False" w579 {
              tunnel: w573 -> [w591 w595]
              tunnel: [w590 w595] -> w578
              tunnel: w577 -> [w594 _]
              tunnel: "Ms to top throttle" -> [w593 _]
              frame False {
                n162 = Divide(x=w594, y=w593) -> (x/y=w592:dbl)
                n163 = Multiply(x=w592, y=w591) -> (x*y=w590:dbl)
              }
              frame True {
              }
            }
            n164 = Greater Or Equal?(x=w581, y=w583) -> (x >= y?=w584:bool)
            n165 = Select(t=2, s=w584, f=1) -> (s? t:f=w588:i32)
          }
          frame 2 {
            n166 = Unbundle By Name(w602) -> ("FusedHeading.Heading"=w601:dbl)
          }
        }
        n167 = call "Drive Straight Pigeon Direct.vi"("D Gain"=5e-05, "P Gain"=0.0725, "Max Corrective Throttle"=1.0, "Target angle"=w536, "Throttle"=w553, "Get All"=w538) -> ("Left Motor Value"=w548:dbl, "Right Motor Value"=w554:dbl)  [unwired: 4 in]
        n168 = feedback-in #14(w552) -> ()
        n169 = Negate(x=w554) -> (-x=w549:dbl)
        n170 = feedback-in #15(w561) -> ()
        n171 = feedback-in #16(w537) -> ()
        n172 = Select(t=w564, s=w562, f=4) -> (s? t:f=w565:i32)
      }
      frame 5 {
        w612 = 0.0 ("%VBus")
        w617 = WPI_CANTalonSRX_APIControlMode."Percent VBus" ("Control Mode")
        # "Shoot for time"
        n173 = Multiply(x=w619, y=1000.0) -> (x*y=w620:dbl)
        n174 = feedback #17() -> (w621:u32)  [unwired: 1 in]
        n175 = feedback #18(0 ("f")) -> (w624:i32)
        n176 = case shown="0, Default" w624 {
          tunnel: [FALSE FALSE TRUE] -> w627
          tunnel: [1 ("f") w646 0 ("f")] -> w626
          tunnel: w621 -> [_ w640 _]
          tunnel: [FALSE TRUE TRUE] -> w622
          tunnel: w620 -> [_ w641 _]
          tunnel: [0.0 8600.0 0.0] -> w613
          tunnel: [bool[] [FALSE] ("Buttons") bool[] [TRUE] ("Buttons") bool[] [FALSE] ("Buttons")] -> w608
          tunnel: [0.0 1.0 0.0] -> w607
          frame 0, Default {
          }
          frame 1 {
            n177 = Greater Or Equal?(x=w640, y=w641) -> (x >= y?=w642:bool)
            n178 = Select(t=2, s=w642, f=1) -> (s? t:f=w646:i32)
          }
          frame 2 {
          }
        }
        n179 = call "ms.vi"("Reset"=w622) -> ("millisecond"=w623:u32)
        n180 = feedback-in #17(w623) -> ()
        n181 = feedback-in #18(w626) -> ()
        n182 = Unbundle By Name(w609) -> ("Sensor Velocity"=w616:dbl)
        n183 = call "Shooter Control and protect.vi"("Auto Reset Delay (ms)"=w612, "Target RPM"=w613, "%VBus"=w612, "Talon Status"=w609) -> ("Output"=w610:dbl, "Control Mode"=w611:T17)  [unwired: 5 in, 1 out]
        n184 = Select(t=w629, s=w627, f=4) -> (s? t:f=w630:i32)
        n185 = call "FeederControl.vi"("Target RPM"=w613, "RPM"=w616, "Buttons"=w608) -> ("Output"=w614:dbl, "Control Mode"=w615:T17)  [unwired: 7 in]
      }
      frame 50 {
        # "Custom Operation"
      }
      frame 51 {
        w657 = 51 ("f")
        w670 = 0 ("f")
        # "Prevent unintentional repeating"
        # "Increment and mannage index"
        # "Saves the Sequence to be run"
        # "Checks if this is the first time the case has been called since start"
        # "Custom Sequence Iterater"
        n186 = Equal To 0?(x=w666) -> (x = 0?=w658:bool)
        n187 = feedback #19(w663) -> (w664:dbl)
        n188 = Select(t=w663, s=w658, f=w664) -> (s? t:f=w662:dbl)
        n189 = feedback-in #19(w662) -> ()
        n190 = case shown="3" w662 {
          tunnel: [w675 "Custom Sequence 1" "Custom Sequence 2" w685] -> w661
          frame 0, Default {
            w675 = cluster{"Values":dbl[], "Operation":u16[]} {"Values"=[0.0], "Operation"=[1000]}  # Custom Sequence Constant
            # "This constant contains a\nsequence that instantly ends\nthe auto."
          }
          frame 1 {
          }
          frame 2 {
          }
          frame 3 {
            w683 = cluster{"Values":dbl[], "Operation":u16[]} {"Values"=[0.0], "Operation"=[1000]}  # Custom Sequence Constant
            n191 = Unbundle By Name(w683) -> ("Operation"=w681:u16[], "Values"=w682:dbl[])
            n192 = call-poly <vilib>:"NT Read Value.vi"("Default Value"=w682, "Name"="Values") -> ("Numeric Array"=w684:dbl[])  [unwired: 8 in, 1 out]
            n193 = call-poly <vilib>:"NT Read Value.vi"("Default Value"=w681, "Name"="Operations") -> ("Numeric Array"=w680:dbl[])  [unwired: 8 in, 1 out]
            n194 = Bundle By Name(cluster=w683, "Operation"=w680, "Values"=w684) -> (w685:cluster{"Values":dbl[], "Operation":u16[]})
          }
        }
        n195 = Unbundle By Name(w661) -> ("Operation"=w674:u16[], "Values"=w673:dbl[])
        n196 = feedback #20(w670) -> (w672:i32)
        n197 = Increment(x=w672) -> (x+1=w668:i32)
        n198 = Select(t=w670, s=w658, f=w668) -> (s? t:f=w669:i32)
        n199 = feedback-in #20(w669) -> ()
        n200 = Index Array(array=w674, index=w672) -> (element=w667:u16)
        n201 = Index Array(array=w673, index=w672) -> (element=w671:dbl)
        n202 = Equal To 0?(x=w667) -> (x = 0?=w660:bool)
        n203 = Or(x=w658, y=w660) -> (x .or. y?=w659:bool)
        n204 = Select(t=w657, s=w659, f=w667) -> (s? t:f=w665:i32)
      }
      frame 100 {
        # "BOILER SIDE\nGo to intersect with peg"
      }
      frame 101 {
        # "Turn to face peg"
        n205 = Unbundle By Name(w695) -> ("FusedHeading.Heading"=w694:dbl)
        n206 = call <vilib>:"NetComm_getAllianceStation.vi"() -> ("Alliance Station"=w689:T18)  [unwired: 10 in, 1 out]
        n207 = Negate(x=w694) -> (-x=w693:dbl)
        n208 = case shown="\"Red 1\"..\"Red 3\"" w689 {
          tunnel: [w698 w700] -> w691
          tunnel: 60.0 -> [w698 w699]
          frame "Blue 1".."Blue 3", Default {
          }
          frame "Red 1".."Red 3" {
            n209 = Negate(x=w699) -> (-x=w700:dbl)
          }
        }
        n210 = Add(x=w691, y=w693) -> (x+y=w692:dbl)
      }
      frame 102 {
        # "Turn to face peg with vision"
      }
      frame 103 {
        # "Approach peg"
      }
      frame 104 {
        # "Eject and back away from peg"
      }
      frame 105 {
        # "Turn to face center"
        n211 = Unbundle By Name(w711) -> ("FusedHeading.Heading"=w710:dbl)
      }
      frame 106 {
        # "Drive to center"
      }
      frame 200 {
        # "FEEDER SIDE\nDrive away from wall"
      }
      frame 201 {
        # "Turn to face gear"
        n212 = call <vilib>:"NetComm_getAllianceStation.vi"() -> ("Alliance Station"=w720:T18)  [unwired: 10 in, 1 out]
        n213 = Unbundle By Name(w724) -> ("FusedHeading.Heading"=w725:dbl)
        n214 = case shown="\"Red 1\"..\"Red 3\"" w720 {
          tunnel: [w729 w731] -> w722
          tunnel: 60.0 -> [w729 w730]
          frame "Blue 1".."Blue 3", Default {
          }
          frame "Red 1".."Red 3" {
            n215 = Negate(x=w730) -> (-x=w731:dbl)
          }
        }
        n216 = Negate(x=w725) -> (-x=w723:dbl)
        n217 = Add(x=w722, y=w723) -> (x+y=w726:dbl)
      }
      frame 202 {
        # "Turn to face with vision"
      }
      frame 203 {
        # "Approach Peg"
      }
      frame 204 {
        # "Back Away from gear"
      }
      frame 205 {
        # "Face center"
        n218 = Unbundle By Name(w744) -> ("FusedHeading.Heading"=w741:dbl)
      }
      frame 206 {
        # "Drive to center"
      }
      frame 300 {
        # "CENTER\nApproach Gear"
      }
      frame 301 {
        # "Eject and back away"
      }
      frame 302 {
        # "Turn towards boiler"
        n219 = call <vilib>:"NetComm_getAllianceStation.vi"() -> ("Alliance Station"=w758:T18)  [unwired: 10 in, 1 out]
        n220 = case shown="\"Red 1\"..\"Red 3\"" w758 {
          tunnel: [w759 w761] -> w756
          tunnel: 0.0 -> [w759 w760]
          frame "Blue 1".."Blue 3", Default {
          }
          frame "Red 1".."Red 3" {
            n221 = Negate(x=w760) -> (-x=w761:dbl)
          }
        }
      }
      frame 400 {
        # "Dance lol"
      }
      frame 401 {
        # "lol..."
      }
      frame 402 {
        n222 = Unbundle By Name(w770) -> ("FusedHeading.Heading"=w774:dbl)
        n223 = Negate(x=w774) -> (-x=w772:dbl)
        n224 = Add(x=-90.0 ("Value to pass"), y=w772) -> (x+y=w771:dbl)
      }
      frame 403 {
        n225 = Unbundle By Name(w777) -> ("FusedHeading.Heading"=w781:dbl)
        n226 = Negate(x=w781) -> (-x=w779:dbl)
        n227 = Add(x=90.0 ("Value to pass"), y=w779) -> (x+y=w778:dbl)
      }
      frame 500 {
      }
      frame 1000, Default {
        # "Finished"
      }
      frame 1001 {
        w789 = WPI_CANTalonSRX_APIControlMode."Motion Magic" ("Control Mode")
        w790 = 0.0 ("Sensor Position")
        # "Finished Hold Position"
        n228 = Not Equal?(x=w803, y=1001) -> (x != y?=w794:bool)
        n229 = First Call?() -> (First Call?: T/F=w793:bool)
        n230 = Or(x=w794, y=w793) -> (x .or. y?=w795:bool)
        n231 = feedback #21(w790) -> (w798:dbl)
        n232 = feedback #22(w790) -> (w799:dbl)
        n233 = case shown="False" w795 {
          tunnel: w801 -> [_ w813]
          tunnel: w800 -> [_ w812]
          tunnel: w799 -> [w808 _]
          tunnel: [w808 w811] -> w797
          tunnel: w798 -> [w809 _]
          tunnel: [w809 w810] -> w796
          frame False {
            # "maintain positions"
          }
          frame True {
            # "Save positions"
            n234 = Unbundle By Name(w813) -> ("Sensor Position"=w811:dbl)
            n235 = Unbundle By Name(w812) -> ("Sensor Position"=w810:dbl)
          }
        }
        n236 = feedback-in #21(w796) -> ()
        n237 = feedback-in #22(w797) -> ()
      }
    }
    n238 = call <vilib>:"CTRE_CANTalonSRX_ConfigMotionMagic.vi"("error in (no error)"=w137, "Max Acceleration"=w122, "Cruise Velocity"=w123, "CAN Talon SRX Ref"=w138) -> ("error out"=w135:errorcluster, "CAN Talon SRX Ref Out"=w136:T11)  [unwired: 6 in]
    n239 = call <vilib>:"CTRE_CANTalonSRX_ConfigMotionMagic.vi"("error in (no error)"=w139, "Max Acceleration"=w122, "Cruise Velocity"=w123, "CAN Talon SRX Ref"=w140) -> ("error out"=w133:errorcluster, "CAN Talon SRX Ref Out"=w134:T11)  [unwired: 6 in]
    n240 = case shown="True" "Disable Drive" {
      tunnel: w70 -> [w202 _]
      tunnel: w72 -> [w203 _]
      tunnel: [w203 0.0 ("Sensor Position")] -> w71
      tunnel: [w202 w204] -> w69
      tunnel: w66 -> [w200 _]
      tunnel: w68 -> [w201 _]
      tunnel: [w201 0.0 ("Sensor Position")] -> w67
      tunnel: [w200 w204] -> w65
      frame False {
      }
      frame True {
        w204 = WPI_CANTalonSRX_APIControlMode."Percent VBus" ("Control Mode")
      }
    }
    n241 = feedback-in #2(w154) -> ()
    n242 = feedback-in #3(w79) -> ()
    n243 = feedback-in #4(w159) -> ()
    n244 = Tick Count (ms)() -> (millisecond timer value=w56:u32)
    n245 = call "Auto gear.vi"("Requested Output"=w78, "Requested Control mode"=w77) -> ("Applied Output"=w75:dbl, "Control Mode"=w76:T17)  [unwired: 8 in]
    n246 = Decrement(x=w56) -> (x-1=w55:u32)
    n247 = global read "Robot Global Data.vi" "LED Color"() -> (w59:T5)
    n248 = feedback #23(w55) -> (w142:u32)
    n249 = case shown="False" w132 {
      tunnel: w56 -> [w236 w241]
      tunnel: w142 -> [w237 _]
      tunnel: [w237 w239] -> w143
      tunnel: [w235 TRUE] -> w60
      frame False {
        n250 = Greater Or Equal?(x=w237, y=w236) -> (x >= y?=w235:bool)
      }
      frame True {
        n251 = Add(x=w241, y=u32 750) -> (x+y=w239:u32)
      }
    }
    n252 = feedback-in #23(w143) -> ()
    n253 = Select(t=T5."GREEN", s=w60, f=w59) -> (s? t:f=w53:T5)
    n254 = call-poly <vilib>:"NT Write Value.vi"("Numeric"=w53, "Name"="Color") -> ()  [unwired: 9 in, 1 out]
    n255 = disable-structure shown="Disabled" {
      disable-tunnel: T4."SOLID" ("Display Mode") -> [w199 _]
      disable-tunnel: w53 -> [w197 _]
      frame Disabled {
        n256 = call "Get and Set LED.vi"("Display Mode"=w199, "Color"=w197, "refnum name"="LEDs") -> ()  [unwired: 9 in]
      }
      frame Enabled {
      }
    }
    n257 = call <vilib>:"WPI_CANTalonSRX_ChangeMode.vi"("error in (no error)"=w147, "Output"=w145, "Control Mode"=w146, "CAN Talon SRX Ref"=w148) -> ("error out"=w96:errorcluster, "CAN Talon SRX Ref"=w97:T11)  [unwired: 6 in]
    n258 = call <vilib>:"WPI_CANTalonSRX_ChangeMode.vi"("error in (no error)"=w99, "Output"=w195, "Control Mode"=w194, "CAN Talon SRX Ref"=w100) -> ("error out"=w85:errorcluster, "CAN Talon SRX Ref"=w86:T11)  [unwired: 6 in]
    n259 = call <vilib>:"WPI_CANTalonSRX_ChangeMode.vi"("error in (no error)"=w169, "Output"=w75, "Control Mode"=w76, "CAN Talon SRX Ref"=w168) -> ("error out"=w83:errorcluster, "CAN Talon SRX Ref"=w84:T11)  [unwired: 6 in]
    n260 = call <vilib>:"WPI_CANTalonSRX_ChangeMode.vi"("error in (no error)"=w171, "Output"=w116, "Control Mode"=w117, "CAN Talon SRX Ref"=w170) -> ("error out"=w81:errorcluster, "CAN Talon SRX Ref"=w82:T11)  [unwired: 6 in]
    n261 = call <vilib>:"WPI_CANTalonSRX_ChangeMode.vi"("error in (no error)"=w133, "Output"=w71, "Control Mode"=w69, "CAN Talon SRX Ref"=w134) -> ("error out"=w152:errorcluster, "CAN Talon SRX Ref"=w153:T11)  [unwired: 6 in]
    n262 = call <vilib>:"WPI_CANTalonSRX_ChangeMode.vi"("error in (no error)"=w135, "Output"=w67, "Control Mode"=w65, "CAN Talon SRX Ref"=w136) -> ("error out"=w150:errorcluster, "CAN Talon SRX Ref"=w151:T11)  [unwired: 6 in]
  }
  n263 = call <vilib>:"CTRE_PigeonIMU_SetFusedHeading.vi"("error in (no error)"=w44, "TareType (SetValue)"=w46, "Value"=0.0, "PigeonIMUDevRef 2"=w45) -> ()  [unwired: 6 in, 2 out]
  n264 = while {
    stop <- FALSE stop-if-true
    n265 = Wait (ms)(milliseconds to wait=u32 20) -> ()  [unwired: 1 out]
    n266 = call <vilib>:"WPI_DriverStationReport Robot Code State.vi"("Autonomous"=TRUE) -> ()  [unwired: 10 in, 1 out]
  }
  n267 = call <vilib>:"WPI_CANTalonSRX_SetSensorPosition.vi"("error in (no error)"=w48, "New Sensor Position"=w47, "CAN Talon SRX Ref"=w49) -> ("error out"=w26:errorcluster, "CAN Talon SRX Ref"=w25:T11)  [unwired: 7 in]
  n268 = call <vilib>:"WPI_CANTalonSRX_SetSensorPosition.vi"("error in (no error)"=w50, "New Sensor Position"=w47, "CAN Talon SRX Ref"=w51) -> ("error out"=w28:errorcluster, "CAN Talon SRX Ref"=w27:T11)  [unwired: 7 in]
  n269 = call <vilib>:"WPI_MotorControlRefNum Registry Get.vi"("refnum name"="LeftDrive2") -> ("error out"=w2:errorcluster, "MotorControlDevRef"=w3:T11)  [unwired: 9 in]
  n270 = call <vilib>:"WPI_MotorControlRefNum Registry Get.vi"("refnum name"="RightDrive2") -> ("error out"=w4:errorcluster, "MotorControlDevRef"=w5:T11)  [unwired: 9 in]
  n271 = call <vilib>:"WPI_CANTalonSRX_ConfigBrakeCoast.vi"("error in (no error)"=w2, "Brake / Coast Mode"=w1, "CAN Talon SRX Ref"=w3) -> ()  [unwired: 7 in, 2 out]
  n272 = call <vilib>:"WPI_CANTalonSRX_ConfigBrakeCoast.vi"("error in (no error)"=w4, "Brake / Coast Mode"=w1, "CAN Talon SRX Ref"=w5) -> ()  [unwired: 7 in, 2 out]
  n273 = call <vilib>:"WPI_CANTalonSRX_ConfigBrakeCoast.vi"("error in (no error)"=w23, "Brake / Coast Mode"=WPI_CANTalonSRX_BrakeOverride."No Override", "CAN Talon SRX Ref"=w24) -> ()  [unwired: 7 in, 2 out]
  n274 = call <vilib>:"WPI_CANTalonSRX_ConfigBrakeCoast.vi"("error in (no error)"=w14, "Brake / Coast Mode"=w1, "CAN Talon SRX Ref"=w15) -> ()  [unwired: 7 in, 2 out]
  n275 = call <vilib>:"WPI_CANTalonSRX_ConfigBrakeCoast.vi"("error in (no error)"=w12, "Brake / Coast Mode"=w8, "CAN Talon SRX Ref"=w13) -> ()  [unwired: 7 in, 2 out]
  n276 = call <vilib>:"WPI_CANTalonSRX_ConfigBrakeCoast.vi"("error in (no error)"=w10, "Brake / Coast Mode"=w8, "CAN Talon SRX Ref"=w11) -> ()  [unwired: 7 in, 2 out]
  n277 = call <vilib>:"WPI_CANTalonSRX_ConfigBrakeCoast.vi"("error in (no error)"=w28, "Brake / Coast Mode"=w1, "CAN Talon SRX Ref"=w27) -> ()  [unwired: 7 in, 2 out]
  n278 = call <vilib>:"WPI_CANTalonSRX_ConfigBrakeCoast.vi"("error in (no error)"=w26, "Brake / Coast Mode"=w1, "CAN Talon SRX Ref"=w25) -> ()  [unwired: 7 in, 2 out]
